vi "Is Uniform Boolean Array.vi"(1 "Array":bool[](array[boolean])) -> (0 "Is Uniform Array":bool)   [LabVIEW 2021, in "PMIC Common.lvlib"]
uses:
  PMIC Common.lvlib
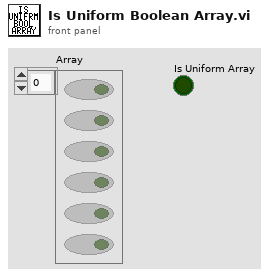
[diagram p1: front panel]
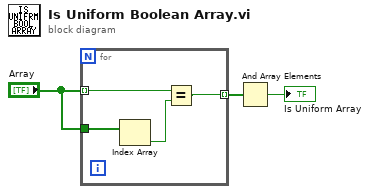
[diagram p0: block diagram]
diagram:
  n1 = for {
    tunnel: "Array" -> [w6] mode=indexing
    tunnel: "Array" -> [w7]
    tunnel: [w4] -> w2 mode=indexing
    n2 = Index Array(array=w7) -> (element=w5:bool)  [unwired: 1 in]
    n3 = Equal?(x=w6, y=w5) -> (x = y?=w4:bool)
  }
  n4 = And Array Elements(Boolean array=w2) -> (logical AND=→"Is Uniform Array":bool)
